vi "SetCalcPar.vi"(4 "Operation Name":string, 6 "InstrPar":T1, 8 "error in (no error)":errorcluster caption="entrée d'erreur (pas d'erreur)", 9 "DataQNames":string[](array[string]), 10 "Calc_Func":T2, 11 "GenData In":refnum<class "Calculations.lvclass"> caption="DNL_LabVIEW Object in") -> (0 "error out":errorcluster caption="sortie d'erreur", 3 "GenData Out":refnum<class "Calculations.lvclass"> caption="DNL_LabVIEW Object out")   [LabVIEW 2019, in "Calculations.lvclass"]
uses:
  Calculations.lvclass
  C:/Programmes Labview/LabScanV1A/DevicesClass/BaseDevice/BaseDevice.lvclass
  DefaultDev_Func.ctl
  Calculations.lvclass/Calculations.ctl
  DevicesClass/BaseDevice/BaseDevice.lvclass/BaseDevice.ctl
  DevicesClass/BaseDevice/Accessor/SetClassEvent.vi
  DevicesClass/BaseDevice/Accessor/SetClassQueue.vi
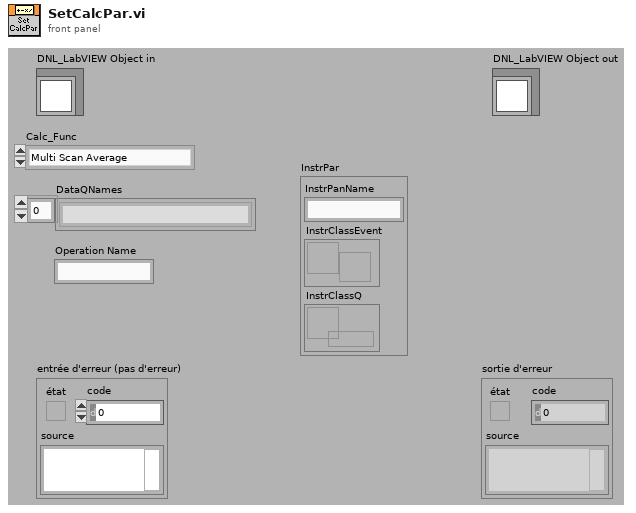
[diagram p1: front panel]
types:
  T1 = cluster{"InstrPanName":string, "InstrClassEvent":refnum<user-event>, "InstrClassQ":refnum<queue>}
  T2 = typedef "Calculations.lvclass/DefaultDev_Func.ctl" = enum16{"Multi Scan Average", "Running Average", "Summ"}
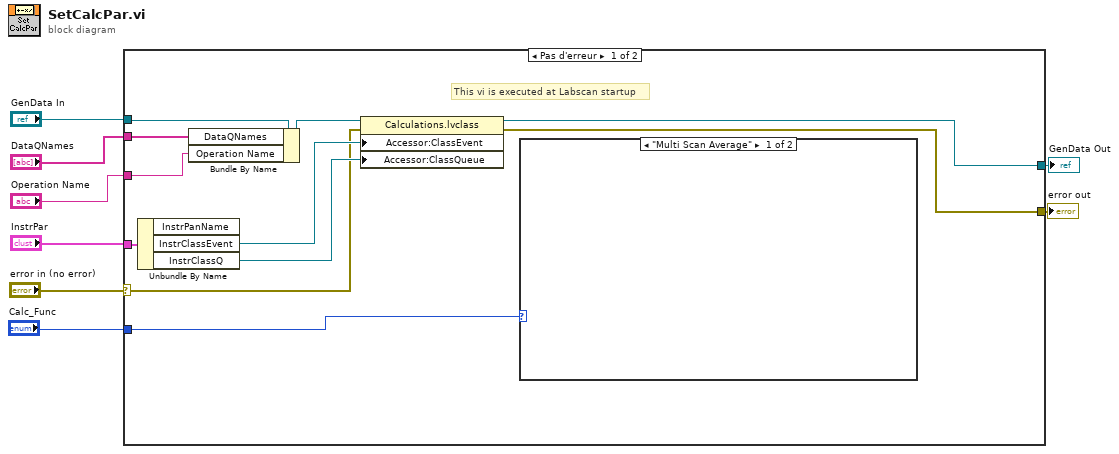
[diagram p0: block diagram]
diagram:
  n1 = case shown="Pas d'erreur" "error in (no error)" {
    selector: "error in (no error)" -> [w11 w21]
    tunnel: [w10 w21] -> w7
    tunnel: "GenData In" -> [w19 w20]
    tunnel: [w14 w20] -> w5
    tunnel: "Calc_Func" -> [w18 _]
    tunnel: "DataQNames" -> [w16 _]
    tunnel: "InstrPar" -> [w15 _]
    tunnel: "Operation Name" -> [w9 _]
    frame No Error {
      # "This vi is executed at Labscan startup"
      n2 = Unbundle By Name(w15) -> ("InstrClassEvent"=w13:refnum<user-event>, "InstrClassQ"=w12:refnum<queue>)  [unwired: 1 out]
      n3 = Bundle By Name(cluster=w19, "DataQNames"=w16, "Operation Name"=w9) -> (w17:refnum<class "Calculations.lvclass">)
      n4 = property class="Calculations.lvclass"(reference=w17, error in=w11, "Accessor:ClassEvent"=w13, "Accessor:ClassQueue"=w12) -> (reference out=w14:refnum<class "Calculations.lvclass">, error out=w10:errorcluster)
      n5 = case shown="\"Multi Scan Average\"" w18 {
        frame "Multi Scan Average" {
        }
        frame Default {
        }
      }
    }
    frame Error {
    }
  }
  "error out" <- w7
  "GenData Out" <- w5
